vi "getFPGA.vi"(11 "ModbusRxDataFIFO in":refnum<class "ModbusRxDataFIFO.lvclass">) -> (2 "FPGA":refnum<class "FPGA.lvclass">, 3 "ModbusRxDataFIFO out":refnum<class "ModbusRxDataFIFO.lvclass">)   [LabVIEW 2016, in "ModbusRxDataFIFO.lvclass"]
uses:
  ModbusRxDataFIFO.lvclass
  FPGA/FPGA.lvclass
  ModbusRxDataFIFO.lvclass/ModbusRxDataFIFO.ctl
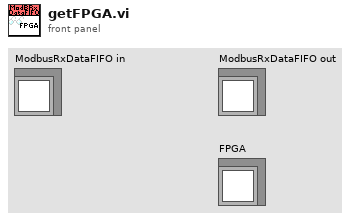
[diagram p1: front panel]
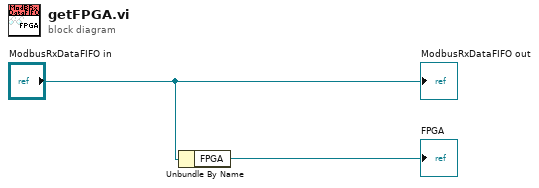
[diagram p0: block diagram]
diagram:
  n1 = Unbundle By Name("ModbusRxDataFIFO in") -> ("FPGA"=→"FPGA":refnum<class "FPGA.lvclass">)
  "ModbusRxDataFIFO out" <- "ModbusRxDataFIFO in"
